vi "local drive robot.vi"() -> ()   [LabVIEW 2018]
uses:
  <vilib>/MakerHub/Xbox-One-Controller/Public/Open First Controller.vi
  <vilib>/MakerHub/Xbox-One-Controller/LMH-Xbox-One-Controller.lvlib
panel:
  in  "Reverse y-axis?":bool=TRUE
  in  "Reverse x-axis?":bool
  in  "Deadband value (0)":i32
  in  "Max controller reading":dbl=29767.0
  in  "deadband limit":i32=3000
  in  "stop":bool
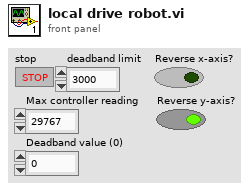
[diagram p1: front panel]
types:
  T1 = typedef "LMH-Xbox-One-Controller.lvlib/Xbox One Controller Ref.ctl" = cluster{"Controller Ref":refnum<k1>, "Event Refnum":refnum<event-registration>, "Worker Ref":refnum<vi>}
  T2 = typedef "LMH-Xbox-One-Controller.lvlib/All Axis Data.ctl" = cluster{"Left Stick":cluster{"X Axis":i32, "Y Axis":i32}, "Right Stick":cluster{"X Axis":i32, "Y Axis":i32}, "Triggers":i32, "D-Pad":T3}
  T3 = typedef "LMH-Xbox-One-Controller.lvlib/DPad Enum.ctl" = enum16{"Idle", "Up", "Up / Right", "Right", "Down / Right", "Down", "Down / Left", "Left", "Up / Left"}
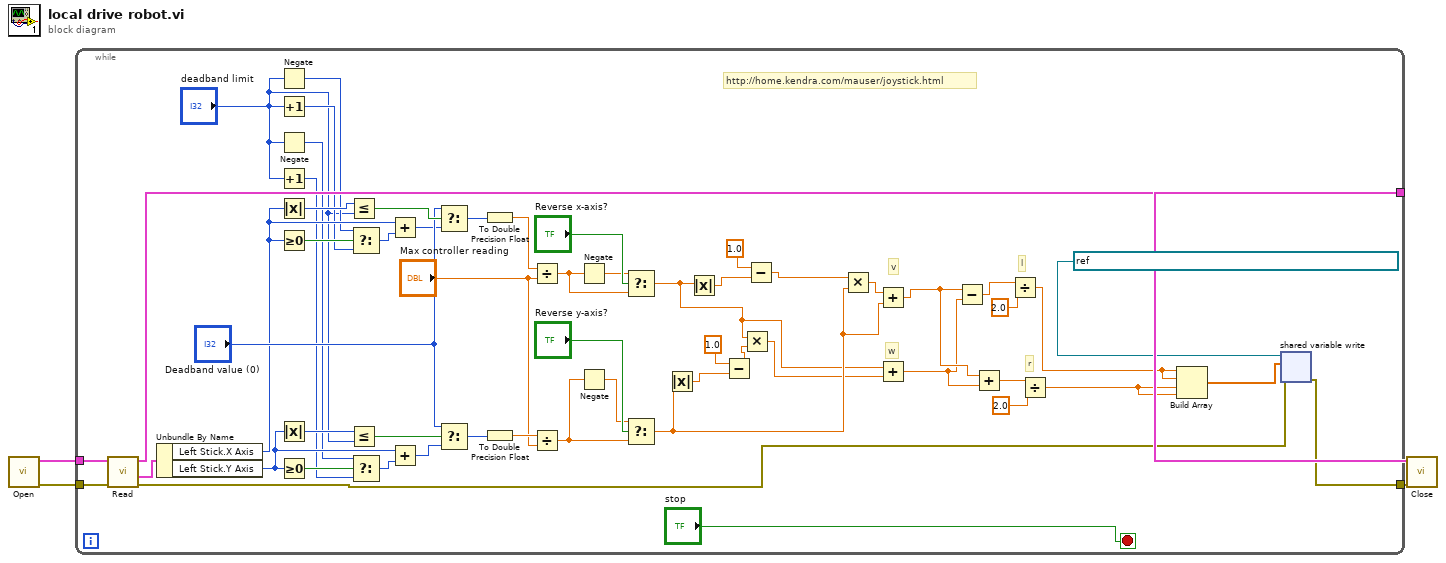
[diagram p0: block diagram]
diagram:
  n1 = call-poly <vilib>:"Open.vi"() -> ("Error Out"=w2:errorcluster, "Xbox One Controller"=w4:T1)  [unwired: 9 in, 1 out]
  n2 = while {
    tunnel: w2 -> [w58]
    tunnel: [w25] -> w1
    tunnel: w4 -> [w60]
    tunnel: [w59] -> w3
    stop <- "stop" stop-if-true
    # "http://home.kendra.com/mauser/joystick.html"
    # "r"
    # "l"
    # "w"
    # "v"
    n3 = call <vilib>:"Read.vi"("Error In"=w58, "Xbox One Controller Ref"=w60) -> ("Error Out"=w26:errorcluster, "All Axis"=w57:T2, "Xbox One Controller Ref"=w59:T1)  [unwired: 6 in, 1 out]
    n4 = Unbundle By Name(w57) -> ("Left Stick.X Axis"=w47:i32, "Left Stick.Y Axis"=w43:i32)
    n5 = Negate(x="deadband limit") -> (-x=w37:i32)
    n6 = Increment(x="deadband limit") -> (x+1=w36:i32)
    n7 = Negate(x="deadband limit") -> (-x=w35:i32)
    n8 = Increment(x="deadband limit") -> (x+1=w34:i32)
    n9 = Absolute Value(x=w47) -> (abs(x)=w52:i32)
    n10 = Greater Or Equal To 0?(x=w47) -> (x >= 0?=w48:bool)
    n11 = Absolute Value(x=w43) -> (abs(x)=w51:i32)
    n12 = Greater Or Equal To 0?(x=w43) -> (x >= 0?=w45:bool)
    n13 = Less Or Equal?(x=w52, y="deadband limit") -> (x <= y?=w54:bool)
    n14 = Less Or Equal?(x=w51, y="deadband limit") -> (x <= y?=w55:bool)
    n15 = Select(t=w37, s=w48, f=w36) -> (s? t:f=w46:i32)
    n16 = Select(t=w35, s=w45, f=w34) -> (s? t:f=w44:i32)
    n17 = Add(x=w47, y=w46) -> (x+y=w50:i32)
    n18 = Add(x=w43, y=w44) -> (x+y=w49:i32)
    n19 = Select(t="Deadband value (0)", s=w54, f=w50) -> (s? t:f=w42:i32)
    n20 = Select(t="Deadband value (0)", s=w55, f=w49) -> (s? t:f=w41:i32)
    n21 = To Double Precision Float(number=w42) -> (double precision float=w40:dbl)
    n22 = To Double Precision Float(number=w41) -> (double precision float=w39:dbl)
    n23 = Divide(x=w40, y="Max controller reading") -> (x/y=w30:dbl)
    n24 = Divide(x=w39, y="Max controller reading") -> (x/y=w28:dbl)
    n25 = Negate(x=w30) -> (-x=w29:dbl)
    n26 = Negate(x=w28) -> (-x=w27:dbl)
    n27 = Select(t=w29, s="Reverse x-axis?", f=w30) -> (s? t:f=w14:dbl)
    n28 = Select(t=w27, s="Reverse y-axis?", f=w28) -> (s? t:f=w17:dbl)
    n29 = Absolute Value(x=w17) -> (abs(x)=w19:dbl)
    n30 = Absolute Value(x=w14) -> (abs(x)=w22:dbl)
    n31 = Subtract(x=1.0 ("s? t:f"), y=w19) -> (x-y=w16:dbl)
    n32 = Multiply(x=w14, y=w16) -> (x*y=w15:dbl)
    n33 = Subtract(x=1.0 ("s? t:f"), y=w22) -> (x-y=w21:dbl)
    n34 = Multiply(x=w21, y=w17) -> (x*y=w20:dbl)
    n35 = Add(x=w20, y=w17) -> (x+y=w11:dbl)
    n36 = Add(x=w14, y=w15) -> (x+y=w10:dbl)
    n37 = Subtract(x=w11, y=w10) -> (x-y=w13:dbl)
    n38 = Add(x=w11, y=w10) -> (x+y=w8:dbl)
    n39 = Divide(x=w13, y=2.0) -> (x/y=w7:dbl)
    n40 = Divide(x=w8, y=2.0) -> (x/y=w6:dbl)
    n41 = Build Array(w7, w7, w6, w6) -> (w5:dbl[])
    n42 = shared-variable-write(refnum<k21> "ni.var.psp://Karims-myRIO/Motor Speeds/Motor Speeds" ("shared variable refnum in"), w26, w5) -> (w25:errorcluster)  [unwired: 1 out]
  }
  n43 = call <vilib>:"Close.vi"("Error In"=w1, "Xbox One Controller Ref"=w3) -> ()  [unwired: 9 in, 1 out]
